vi "environment data insert.vi"(8 "error in (no error)":errorcluster, 10 "环境变量":cluster{"电压":dbl, "室温":dbl, "湿度":dbl}={"电压"=12.0, "室温"=25.0, "湿度"=75.0}, 11 "$GPRMC-message_OUT":T1={"TimeStamp"=timestamp(0 s since 1904-01-01), "Validity"=FALSE, "Latitude"=0.0, "Latitude-Direction"=enum."North", "Longitude"=0.0, "Longitude-Direction"=enum."East", "Speed in knots"=0.0, "True course"=0.0, "Date Stamp"=timestamp(0 s since 1904-01-01), "Magnetic Variation (East/West)"=0.0} {"Magnetic Variation (East/West)" format="%.02f [deg]"; "Date Stamp" format="%<%x>T"; "True course" format="%.02f [deg]"; "Speed in knots" format="%.02f [kts]"; "Longitude" format="%0.4f [long]"; "Latitude" format="%.04f [lat]"; "TimeStamp" format="%<%.2X>T"}) -> (0 "error out":errorcluster)   [LabVIEW 2016, in "AIRMAR WeatherCaster.lvlib"]
uses:
  AIRMAR WeatherCaster.lvlib
  NMEA_GPRMC-data.ctl
  NMEA_LatitudeDirection.ctl
  NMEA_LongitudeDirection.ctl
  <vilib>/addons/database/Auxilliary.llb/DB Tools Column Info.ctl
  <vilib>/addons/database/Auxilliary.llb/DB Tools DataTypes.ctl
  <vilib>/addons/database/NI_Database_API.lvlib
  <vilib>/Utility/VariantDataType/VariantType.lvlib
panel:
  in  "data in":T4
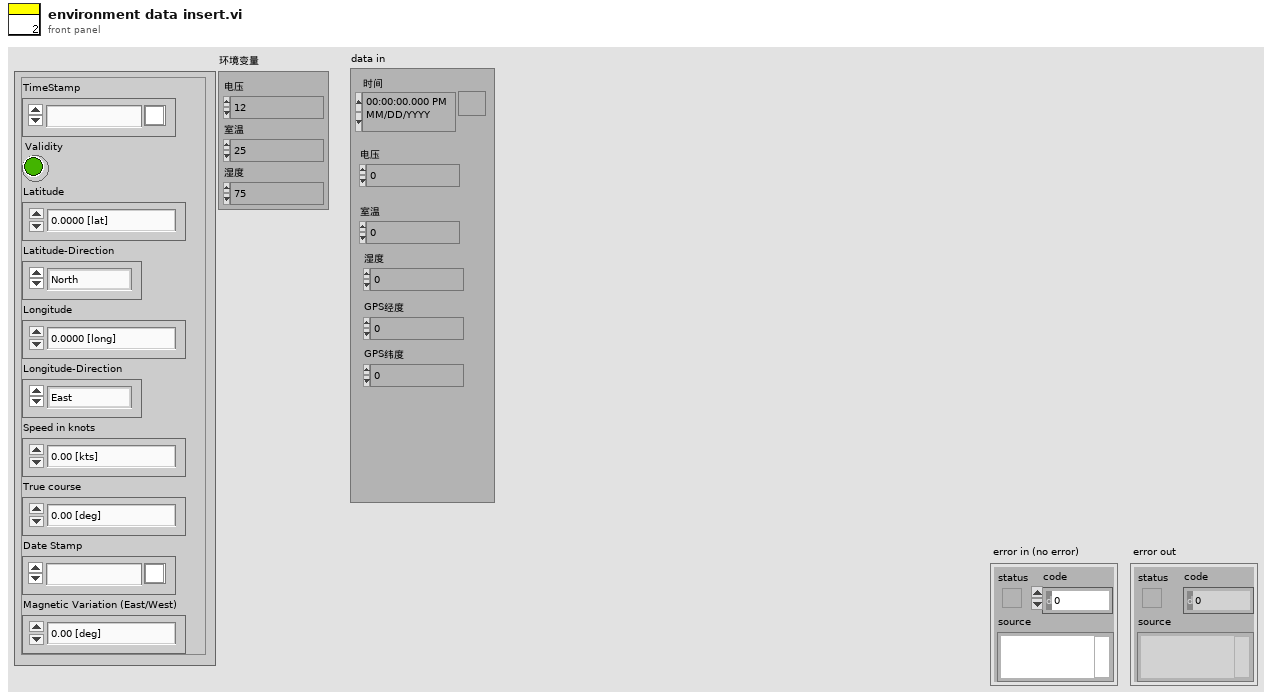
[diagram p1: front panel]
types:
  T1 = typedef "AIRMAR WeatherCaster.lvlib/NMEA_GPRMC-data.ctl" = cluster{"TimeStamp":timestamp, "Validity":bool, "Latitude":dbl, "Latitude-Direction":T2, "Longitude":dbl, "Longitude-Direction":T3, "Speed in knots":dbl, "True course":dbl, "Date Stamp":timestamp, "Magnetic Variation (East/West)":dbl}
  T2 = typedef "AIRMAR WeatherCaster.lvlib/NMEA_LatitudeDirection.ctl" = enum16{"", "North", "South"}
  T3 = typedef "AIRMAR WeatherCaster.lvlib/NMEA_LongitudeDirection.ctl" = enum16{"", "East", "West"}
  T4 = cluster{"时间":timestamp, "电压":dbl, "室温":dbl, "湿度":dbl, "GPS经度":dbl, "GPS纬度":dbl}
  T5 = typedef "NI_Database_API.lvlib/DB Tools Column Info.ctl" = cluster{"column name":string, "data type":T6, "size":i32, "allow null?":bool}
  T6 = typedef "NI_Database_API.lvlib/DB Tools DataTypes.ctl" = enum16{"String", "Long (I32)", "Single (SGL)", "Double (DBL)", "Date/Time", "Binary"}
  T7 = typedef "VariantType.lvlib/Type.ctl" = enum8{"Invalid Type", "Void", "I8", "I16", "I32", "I64", "U8", "U16", "U32", "U64", "Single Float", "Double Float", "Extended Float", "Single Complex", "Double Complex", "Extended Complex", "Enum U8", "Enum U16", "Enum U32", "Enum U64", "Single Float With Unit", "Double Float With Unit", "Extended Float With Unit", "Single Complex with Unit", "Double Complex with Unit", "Extended Complex with Unit", "Boolean", "String", "Path", "Picture", "Tag", "Array", "Cluster", "Variant", "LV Variant", "Waveform", "Timestamp", "Digital Waveform", "Digital Data", "ExpressData", "Refnum", "External Data", "VI", "Poly VI", "LabVIEW Class Instance", "Fixed Point"}
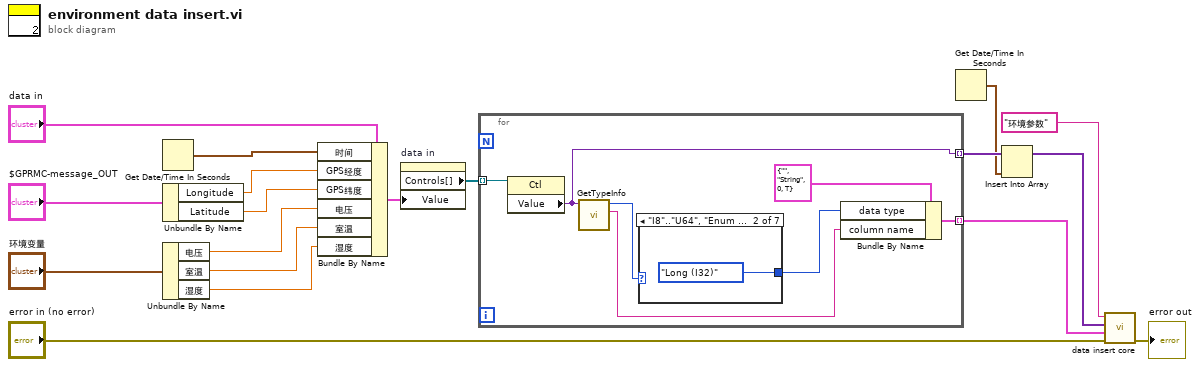
[diagram p0: block diagram]
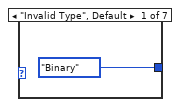
[diagram p2: hidden frame]
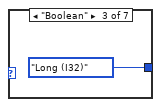
[diagram p3: hidden frame]
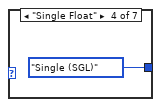
[diagram p4: hidden frame]
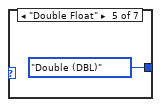
[diagram p5: hidden frame]
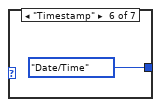
[diagram p6: hidden frame]
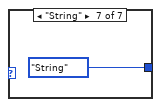
[diagram p7: hidden frame]
diagram:
  n1 = Get Date/Time In Seconds() -> (seconds since 1Jan1904=w9:timestamp)
  n2 = Unbundle By Name("$GPRMC-message_OUT") -> ("Longitude"=w6:dbl, "Latitude"=w5:dbl)
  n3 = Unbundle By Name("环境变量") -> ("电压"=w3:dbl, "室温"=w2:dbl, "湿度"=w1:dbl)
  n4 = Bundle By Name(cluster="data in", "时间"=w9, "GPS经度"=w6, "GPS纬度"=w5, "电压"=w3, "室温"=w2, "湿度"=w1) -> (w8:T4)
  n5 = property on="data in" class="Clust (严格)"("Value"=w8) -> ("Controls[]"=w18:refnum<vi>[])  [unwired: 2 in, 2 out]
  n6 = for {
    tunnel: w18 -> [w25] mode=indexing
    tunnel: [w19] -> w17 mode=indexing
    tunnel: [w20] -> w12 mode=indexing
    n7 = property class="Ctl"(reference=w25) -> ("Value"=w19:variant)  [unwired: 1 in, 2 out]
    n8 = call <vilib>:"GetTypeInfo.vi"("Variant"=w19) -> ("Name"=w23:string, "Type Enum"=w22:T7)  [unwired: 6 in, 3 out]
    n9 = case shown="\"I8\"..\"U64\", \"Enum U8\"..\"Enum U64\"" w22 {
      tunnel: [DB_Tools_DataTypes."Binary" ("data type") DB_Tools_DataTypes."Long (I32)" ("data type") DB_Tools_DataTypes."Long (I32)" ("data type") DB_Tools_DataTypes."Single (SGL)" ("data type") DB_Tools_DataTypes."Double (DBL)" ("data type") DB_Tools_DataTypes."Date/Time" ("data type") DB_Tools_DataTypes."String" ("data type")] -> w21
      frame "Invalid Type", Default {
      }
      frame "I8".."U64", "Enum U8".."Enum U64" {
      }
      frame "Boolean" {
      }
      frame "Single Float" {
      }
      frame "Double Float" {
      }
      frame "Timestamp" {
      }
      frame "String" {
      }
    }
    n10 = Bundle By Name(cluster=T5 {"column name"="", "data type"=enum."String", "size"=0, "allow null?"=TRUE} ("column information"), "data type"=w21, "column name"=w23) -> (w20:T5)
  }
  n11 = Get Date/Time In Seconds() -> (seconds since 1Jan1904=w16:timestamp)
  n12 = Insert Into Array(array=w17, new element=w16) -> (w15:variant[])  [unwired: 1 in]
  n13 = call "data insert core.vi"("error in (no error)"="error in (no error)", "column information"=w12, "data"=w15, "table"="环境参数") -> ("error out"=→"error out":errorcluster)  [unwired: 7 in]
